vi "tentative.vi"() -> ()   [LabVIEW 2017]
uses:
  <vilib>/express/express analysis/Spectral/Block/exnSpectralBlock spectral measurements PSD poly.vi
  <vilib>/express/express analysis/Spectral/Block/exnSpectralBlock spectral measurements PSD DDT.vi
  <vilib>/express/express analysis/Spectral/XNode/ExpressSpectralMeasurementsBlockNode.xnode
panel:
  in  "Nom de périphérique DAQmx classique":tag
  out "DSP filtré":dynamicdata(graph)
  out "Signal":dynamicdata(graph)
  out "DSP":dynamicdata(graph)
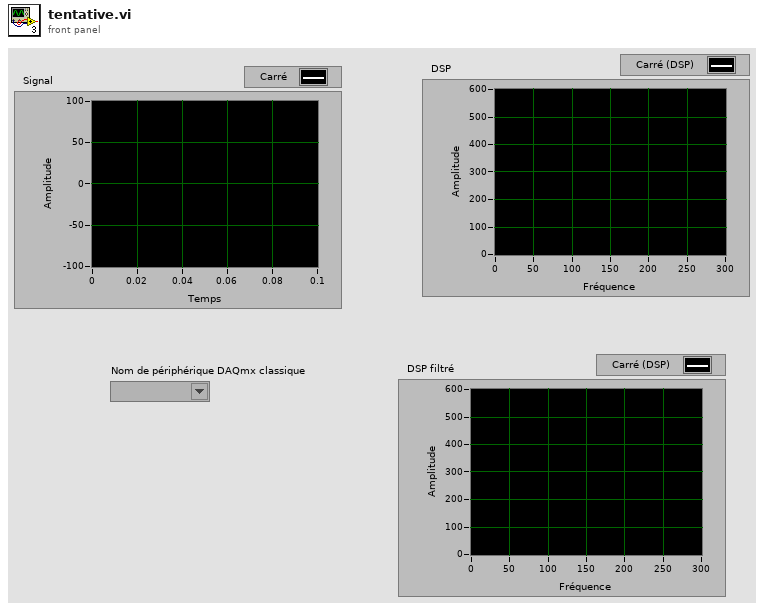
[diagram p1: front panel]
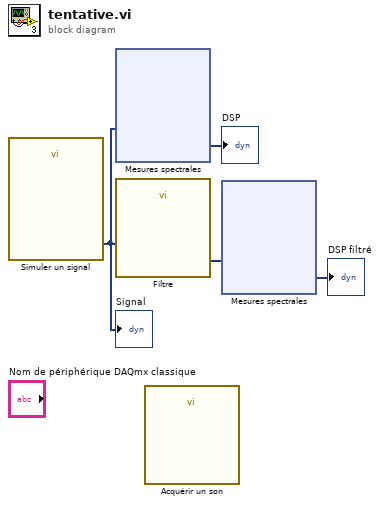
[diagram p0: block diagram]
diagram:
  n1 = call "Simuler un signal"() -> ("Carré"=w2:dynamicdata)  [unwired: 14 in, 1 out]
  "Signal" <- w2
  n2 = xnode "Mesures spectrales"("Signaux"=w2) -> ("DSP"=→"DSP":dynamicdata)  [unwired: 1 in, 1 out]
  n3 = call "Filtre"("Signal"=w2) -> ("Filtered Signal"=w3:dynamicdata)  [unwired: 9 in, 1 out]
  n4 = call "Acquérir un son"() -> ()  [unwired: 18 in, 2 out]
  n5 = xnode "Mesures spectrales"("Signaux"=w3) -> ("DSP"=→"DSP filtré":dynamicdata)  [unwired: 1 in, 1 out]
